vi "CRYRub & Buzz Ethres[k].vi"(9 "Version":i32, 10 "Real matrix":dbl[][](array[numeric])) -> (1 "s[k]":dbl[](array[numeric]), 3 "Ethres[k]":dbl[](array[numeric]))   [LabVIEW 2013]
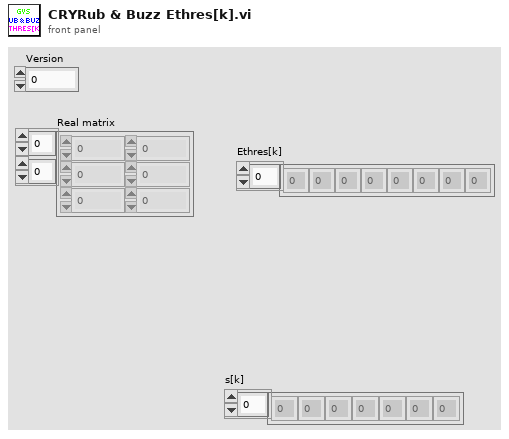
[diagram p1: front panel]
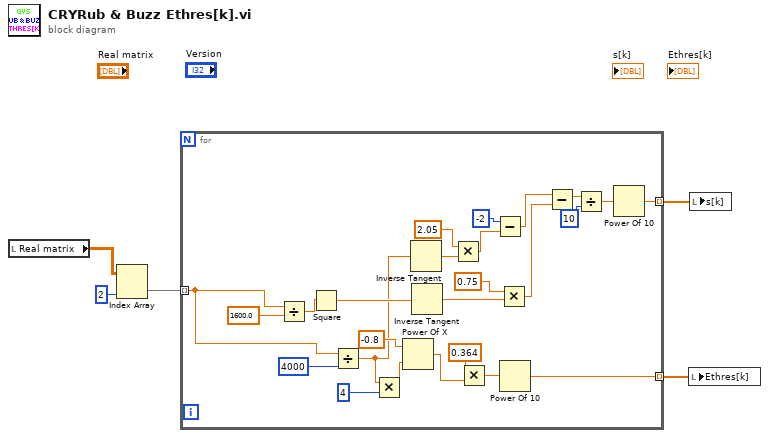
[diagram p0: block diagram]
diagram:
  n1 = local read "Real matrix"() -> (w3:dbl[][])
  n2 = Index Array(array=w3, index (col)=2 ("disabled index (col)")) -> (element=w1:dbl[])  [unwired: 1 in]
  n3 = for {
    tunnel: [w8] -> w5 mode=indexing
    tunnel: [w7] -> w4 mode=indexing
    tunnel: w1 -> [w6] mode=indexing
    n4 = Divide(x=w6, y=1600.0) -> (x/y=w20:dbl)
    n5 = Square(x=w20) -> (x^2=w19:dbl)
    n6 = Divide(x=w6, y=4000) -> (x/y=w10:dbl)
    n7 = Multiply ("Multiply.vi")(x=w10, y=4) -> (x*y=w9:dbl)
    n8 = Power Of X ("Power Of X.vi")(1:w9, 2:-0.8) -> (0:w27:dbl)
    n9 = Inverse Tangent(1:w10) -> (0:w24:dbl)
    n10 = Inverse Tangent(1:w19) -> (0:w12:dbl)
    n11 = Multiply ("Multiply.vi")(x=2.05, y=w24) -> (x*y=w23:dbl)
    n12 = Multiply ("Multiply.vi")(x=0.364, y=w27) -> (x*y=w26:dbl)
    n13 = Subtract ("Subtract.vi")(x=-2, y=w23) -> (x-y=w15:dbl)
    n14 = Multiply ("Multiply.vi")(x=0.75, y=w12) -> (x*y=w14:dbl)
    n15 = Power Of 10(x=w26) -> (10^x=w7:dbl)
    n16 = Subtract ("Subtract.vi")(x=w15, y=w14) -> (x-y=w13:dbl)
    n17 = Divide(x=w13, y=10) -> (x/y=w16:dbl)
    n18 = Power Of 10(x=w16) -> (10^x=w8:dbl)
  }
  n19 = local write "Ethres[k]"(w4) -> ()
  n20 = local write "s[k]"(w5) -> ()
